vi "LogFilter - Check.vi"(8 "Matched Previous?":bool, 10 "Cross CSM Data In":T1, 11 "GlobalLogFilter In":refnum<class "LogFilter.lvclass">) -> (0 "Matched? (Dup)":bool, 2 "Cross CSM Data Out":T1, 3 "GlobalLogFilter.lvclass (Dup)":refnum<class "LogFilter.lvclass">)   [LabVIEW 2017, in "Communicable State Machine.lvlib" / "LogFilter.lvclass"]
uses:
  LogFilter.lvclass
  Typedef/_CSM_GlobalLog_MSG.ctl
  Typedef/_CSM_Response Source Message.ctl
  Typedef/_CSM_GlobalLog_MSG_TYPE.ctl
  LogFilter.lvclass/LogFilter.ctl
  Support/Log State Type.vi
  Communicable State Machine.lvlib
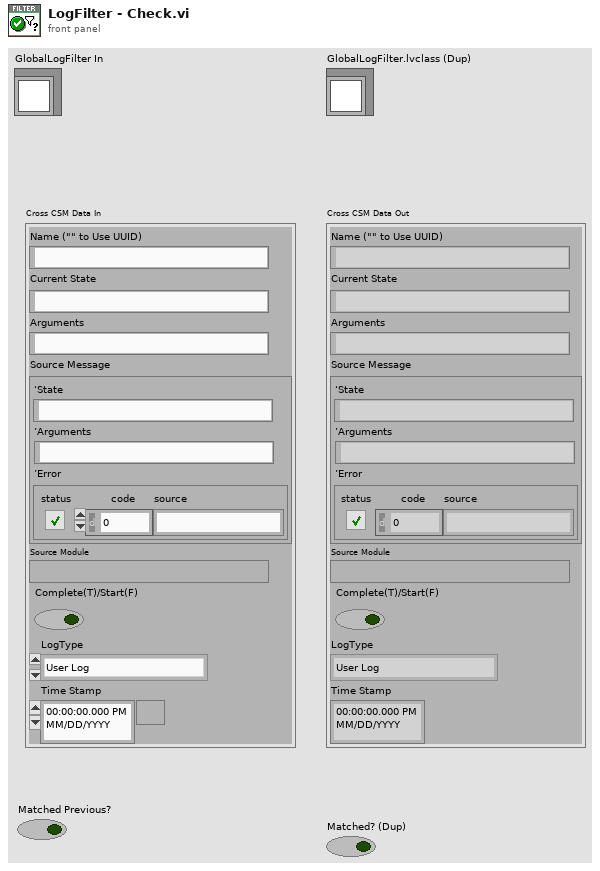
[diagram p1: front panel]
types:
  T1 = typedef "Communicable State Machine.lvlib/_CSM_GlobalLog_MSG.ctl" = cluster{"Name (\"\" to Use UUID)":string, "Current State":string, "Arguments":string, "Source Message":T2, "Source Module":string, "Complete(T)/Start(F)":bool, "LogType":T3, "Time Stamp":timestamp}
  T2 = typedef "Communicable State Machine.lvlib/_CSM_Response Source Message.ctl" = cluster{"‘State":string, "’Arguments":string, "’Error":errorcluster}
  T3 = typedef "Communicable State Machine.lvlib/_CSM_GlobalLog_MSG_TYPE.ctl" = enum16{"User Log", "State Change", "Status", "Interrupt", "Register", "Unregister", "Error Log", "Module Created", "Module Destroyed", "Async Message", "No-Rep Async Message", "Sync Message", "AsyncMsg Complete", "SyncMsg Complete"}
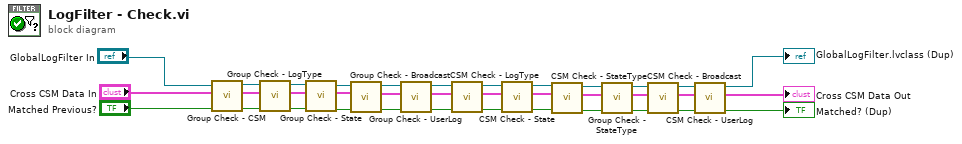
[diagram p0: block diagram]
diagram:
  n1 = call "Group Check - CSM.vi"("Matched Previous?"="Matched Previous?", "Cross CSM Data (In)"="Cross CSM Data In", "GlobalLogFilter.lvclass"="GlobalLogFilter In") -> ("Matched? (Dup)"=w30:bool, "Cross CSM Data"=w29:T1, "GlobalLogFilter.lvclass (Dup)"=w28:refnum<class "LogFilter.lvclass">)  [unwired: 6 in]
  n2 = call "Group Check - LogType.vi"("Matched Previous?"=w30, "Cross CSM Data (In)"=w29, "GlobalLogFilter.lvclass"=w28) -> ("Matched? (Dup)"=w36:bool, "Cross CSM Data"=w32:T1, "GlobalLogFilter.lvclass (Dup)"=w35:refnum<class "LogFilter.lvclass">)  [unwired: 6 in]
  n3 = call "Group Check - State.vi"("Matched Previous?"=w36, "Cross CSM Data (In)"=w32, "GlobalLogFilter.lvclass"=w35) -> ("Matched? (Dup)"=w13:bool, "Cross CSM Data"=w14:T1, "GlobalLogFilter.lvclass (Dup)"=w15:refnum<class "LogFilter.lvclass">)  [unwired: 6 in]
  n4 = call "Group Check - Broadcast.vi"("Matched Previous?"=w13, "Cross CSM Data (In)"=w14, "GlobalLogFilter.lvclass"=w15) -> ("Matched? (Dup)"=w12:bool, "Cross CSM Data"=w11:T1, "GlobalLogFilter.lvclass (Dup)"=w10:refnum<class "LogFilter.lvclass">)  [unwired: 6 in]
  n5 = call "Group Check - UserLog.vi"("Matched Previous?"=w12, "Cross CSM Data (In)"=w11, "GlobalLogFilter.lvclass"=w10) -> ("Matched? (Dup)"=w9:bool, "Cross CSM Data"=w8:T1, "GlobalLogFilter.lvclass (Dup)"=w7:refnum<class "LogFilter.lvclass">)  [unwired: 6 in]
  n6 = call "CSM Check - LogType.vi"("Matched Previous?"=w9, "Cross CSM Data (In)"=w8, "GlobalLogFilter.lvclass"=w7) -> ("Matched? (Dup)"=w25:bool, "Cross CSM Data"=w27:T1, "GlobalLogFilter.lvclass (Dup)"=w26:refnum<class "LogFilter.lvclass">)  [unwired: 6 in]
  n7 = call "CSM Check - State.vi"("Matched Previous?"=w25, "Cross CSM Data (In)"=w27, "GlobalLogFilter.lvclass"=w26) -> ("Matched? (Dup)"=w19:bool, "Cross CSM Data"=w20:T1, "GlobalLogFilter.lvclass (Dup)"=w21:refnum<class "LogFilter.lvclass">)  [unwired: 6 in]
  n8 = call "CSM Check - StateType.vi"("Matched Previous?"=w19, "Cross CSM Data (In)"=w20, "GlobalLogFilter.lvclass"=w21) -> ("Matched? (Dup)"=w24:bool, "Cross CSM Data"=w23:T1, "GlobalLogFilter.lvclass (Dup)"=w22:refnum<class "LogFilter.lvclass">)  [unwired: 6 in]
  n9 = call "Group Check - StateType.vi"("Matched Previous?"=w24, "Cross CSM Data (In)"=w23, "GlobalLogFilter.lvclass"=w22) -> ("Matched? (Dup)"=w16:bool, "Cross CSM Data"=w17:T1, "GlobalLogFilter.lvclass (Dup)"=w18:refnum<class "LogFilter.lvclass">)  [unwired: 6 in]
  n10 = call "CSM Check - Broadcast.vi"("Matched Previous?"=w16, "Cross CSM Data (In)"=w17, "GlobalLogFilter.lvclass"=w18) -> ("Matched? (Dup)"=w4:bool, "Cross CSM Data"=w5:T1, "GlobalLogFilter.lvclass (Dup)"=w6:refnum<class "LogFilter.lvclass">)  [unwired: 6 in]
  n11 = call "CSM Check - UserLog.vi"("Matched Previous?"=w4, "Cross CSM Data (In)"=w5, "GlobalLogFilter.lvclass"=w6) -> ("Matched? (Dup)"=→"Matched? (Dup)":bool, "Cross CSM Data"=→"Cross CSM Data Out":T1, "GlobalLogFilter.lvclass (Dup)"=→"GlobalLogFilter.lvclass (Dup)":refnum<class "LogFilter.lvclass">)  [unwired: 6 in]
